vi "Available Workers.vi"(7 "Refresh? (F)":bool) -> (2 "Variants":cluster{"Variants":string[]}[](array[cluster]), 3 "Available Workers":string[](array[string]))   [LabVIEW 2020, in "FlexBlocks.lvlib"]
uses:
  FlexBlocks.lvlib
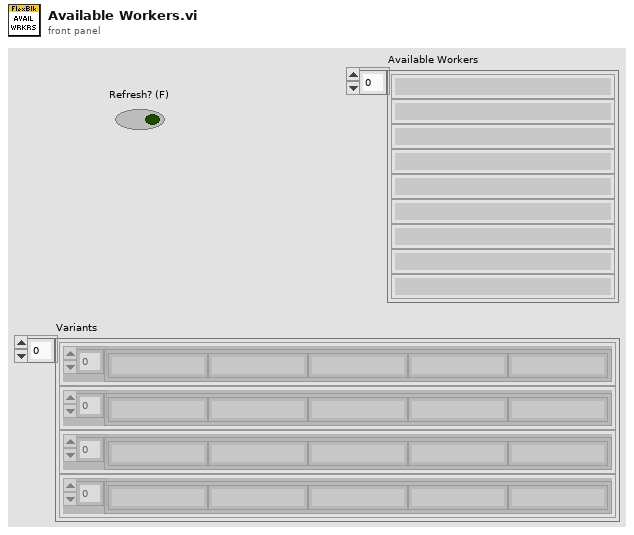
[diagram p1: front panel]
types:
  T1 = typedef "FlexBlocks.lvlib/Paths.ctl" = cluster{"FlexBlocks":path, "Workers Root":path, "Specialized Editors":path, "Worker Template":path, "Editor Template":path, "Express Template":path}
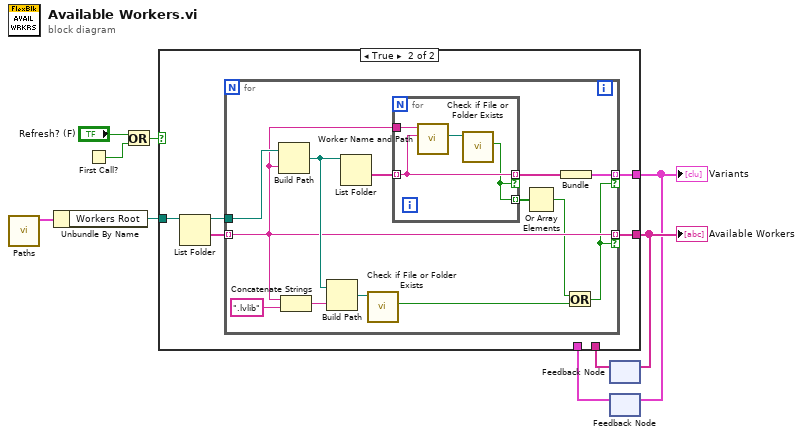
[diagram p0: block diagram]
diagram:
  n1 = call "Paths.vi"() -> ("Paths"=w2:T1)  [unwired: 11 in]
  n2 = Unbundle By Name(w2) -> ("Workers Root"=w1:path)
  n3 = First Call?() -> (First Call?: T/F=w8:bool)
  n4 = Or(x="Refresh? (F)", y=w8) -> (x .or. y?=w7:bool)
  n5 = feedback #1() -> (w5:string[])  [unwired: 1 in]
  n6 = feedback #2() -> (w3:cluster{string[]}[])  [unwired: 1 in]
  n7 = case shown="True" w7 {
    tunnel: w1 -> [_ w16]
    tunnel: [w11 w13] -> w6
    tunnel: [w10 w12] -> w4
    tunnel: w5 -> [w11 _]
    tunnel: w3 -> [w10 _]
    frame False {
    }
    frame True {
      n8 = List Folder(path=w16) -> (path out=w14:path, folder names=w15:string[])  [unwired: 3 in, 2 out]
      n9 = for {
        tunnel: w15 -> [w22] mode=indexing
        tunnel: w14 -> [w29]
        tunnel: [w22] -> w13 mode=indexing if=w17
        tunnel: [w20] -> w12 mode=indexing if=w17
        n10 = Build Path(base path=w29, name or relative path=w22) -> (appended path=w25:path)
        n11 = Concatenate Strings(w22, ".lvlib" ("string")) -> (w27:string)
        n12 = Build Path(base path=w25, name or relative path=w27) -> (appended path=w26:path)
        n13 = List Folder(path=w25) -> (folder names=w23:string[])  [unwired: 3 in, 3 out]
        n14 = call <vilib>:"Check if File or Folder Exists.vi"("path"=w26) -> ("file or folder exists?"=w24:bool)  [unwired: 8 in, 2 out]
        n15 = for {
          tunnel: w23 -> [w31] mode=indexing
          tunnel: w22 -> [w33]
          tunnel: [w31] -> w21 mode=indexing if=w30
          tunnel: [w30] -> w19 mode=indexing
          n16 = call "Worker Name and Path.vi"("Variant"=w31, "Worker"=w33) -> ("Path"=w32:path)  [unwired: 6 in, 3 out]
          n17 = call <vilib>:"Check if File or Folder Exists.vi"("path"=w32) -> ("file or folder exists?"=w30:bool)  [unwired: 8 in, 2 out]
        }
        n18 = Or Array Elements(Boolean array=w19) -> (logical OR=w18:bool)
        n19 = Bundle(w21) -> (w20:cluster{string[]})  [unwired: 1 in]
        n20 = Or(x=w18, y=w24) -> (x .or. y?=w17:bool)
      }
    }
  }
  "Available Workers" <- w6
  "Variants" <- w4
  n21 = feedback-in #1(w6) -> ()
  n22 = feedback-in #2(w4) -> ()
